vi "SUB_FindSpecificHEXString.vi"(3 "Find this String":string, 5 "String data":string) -> (0 "before \"; \" string":string, 2 "Found":bool)   [LabVIEW 2011]
panel:
  out "after substring":string
  out "match substring":string
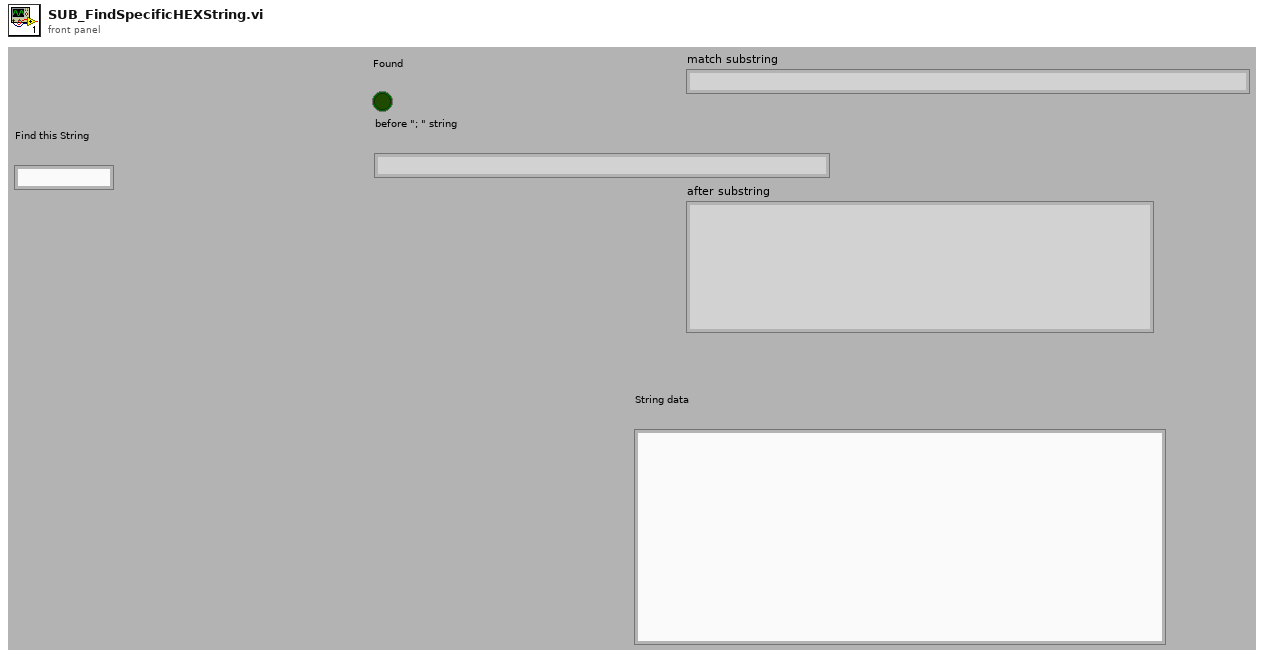
[diagram p1: front panel]
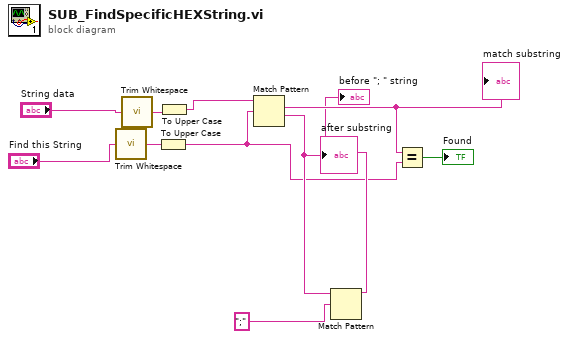
[diagram p0: block diagram]
diagram:
  n1 = call <vilib>:"Trim Whitespace.vi"("string"="Find this String") -> ("trimmed string"=w2:string)  [unwired: 1 in]
  n2 = call <vilib>:"Trim Whitespace.vi"("string"="String data") -> ("trimmed string"=w4:string)  [unwired: 1 in]
  n3 = To Upper Case(1:w2) -> (0:w1:string)
  n4 = To Upper Case(1:w4) -> (0:w3:string)
  n5 = Match Pattern(string=w3, regular expression=w1) -> (match substring=w9:string, after substring=w11:string)  [unwired: 1 in, 2 out]
  "match substring" <- w9
  "after substring" <- w11
  n6 = Match Pattern(string=w11, regular expression=";") -> (before substring=→"before \"; \" string":string)  [unwired: 1 in, 3 out]
  n7 = Equal?(x=w9, y=w1) -> (x = y?=→"Found":bool)
